vi "Init Nav Panels.vi"(8 "error in (no error)":errorcluster, 11 "App in":refnum<class "App.lvclass">) -> (0 "error out":errorcluster, 3 "App out":refnum<class "App.lvclass">)   [LabVIEW 2020, in "PicoG-App.lvlib" / "App.lvclass"]
uses:
  App.lvclass
  <vilib>/IlluminatedG/IG OOPanel/OOPanel/Manager/Manager.lvclass
  AppListPanel/AppListPanel.lvclass
  DeviceListPanel/DeviceListPanel.lvclass
  PlatformListPanel/PlatformListPanel.lvclass
  C:/Program Files (x86)/National Instruments/LabVIEW 2020/vi.lib/IlluminatedG/IG OOPanel/OOPanel/Panel/Panel.lvclass
  C:/dev/Vireo/PicoG/PicoG-App/AppListPanel/AppListPanel.lvclass
  C:/dev/Vireo/PicoG/PicoG-App/PlatformListPanel/PlatformListPanel.lvclass
  C:/dev/Vireo/PicoG/PicoG-App/DeviceListPanel/DeviceListPanel.lvclass
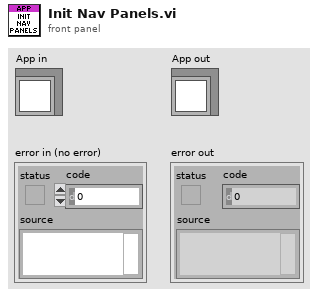
[diagram p1: front panel]
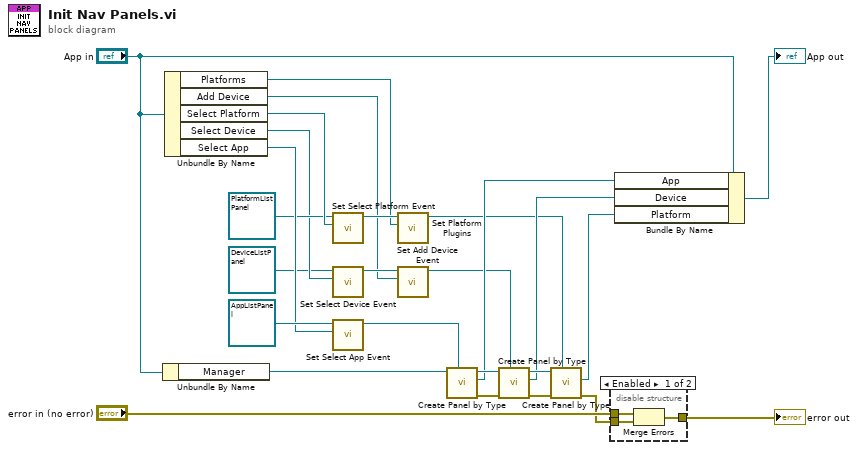
[diagram p0: block diagram]
diagram:
  n1 = Unbundle By Name("App in") -> ("Manager"=w13:refnum<class "Manager.lvclass">)
  n2 = Unbundle By Name("App in") -> ("Platforms"=w1:refnum<class "PlatformPluginManager.lvclass">, "Add Device"=w3:refnum<user-event>, "Select Platform"=w26:refnum<user-event>, "Select Device"=w6:refnum<user-event>, "Select App"=w16:refnum<user-event>)
  n3 = call "Set Select Platform Event.vi"("Select Platform"=w26, "PlatformListPanel in"=refnum<class "PlatformListPanel.lvclass"> refnum ("PicoG-App.lvlib:PlatformListPanel.lvclass")) -> ("PlatformListPanel out"=w8:refnum<class "PlatformListPanel.lvclass">)  [unwired: 8 in, 1 out]
  n4 = call "Set Select Device Event.vi"("Select Device"=w6, "DeviceListPanel in"=refnum<class "DeviceListPanel.lvclass"> refnum ("PicoG-App.lvlib:DeviceListPanel.lvclass")) -> ("DeviceListPanel out"=w4:refnum<class "DeviceListPanel.lvclass">)  [unwired: 8 in, 1 out]
  n5 = call "Set Select App Event.vi"("Select App"=w16, "AppListPanel in"=refnum<class "AppListPanel.lvclass"> refnum ("PicoG-App.lvlib:AppListPanel.lvclass")) -> ("AppListPanel out"=w7:refnum<class "AppListPanel.lvclass">)  [unwired: 8 in, 1 out]
  n6 = call "Set Platform Plugins.vi"("Platform Plugins"=w1, "PlatformListPanel in"=w8) -> ("PlatformListPanel out"=w18:refnum<class "PlatformListPanel.lvclass">)  [unwired: 8 in, 1 out]
  n7 = call "Set Add Device Event.vi"("Add Device"=w3, "DeviceListPanel in"=w4) -> ("DeviceListPanel out"=w2:refnum<class "DeviceListPanel.lvclass">)  [unwired: 8 in, 1 out]
  n8 = call <vilib>:"Create Panel by Type.vi"("Panel Type"=w7, "Manager in"=w13) -> ("error out"=w12:errorcluster, "Panel"=w19:refnum<class "AppListPanel.lvclass">, "Manager out"=w24:refnum<class "Manager.lvclass">)  [unwired: 7 in]
  n9 = call <vilib>:"Create Panel by Type.vi"("Panel Type"=w2, "error in (no error)"=w12, "Manager in"=w24) -> ("error out"=w11:errorcluster, "Panel"=w20:refnum<class "DeviceListPanel.lvclass">, "Manager out"=w23:refnum<class "Manager.lvclass">)  [unwired: 6 in]
  n10 = call <vilib>:"Create Panel by Type.vi"("Panel Type"=w18, "error in (no error)"=w11, "Manager in"=w23) -> ("error out"=w9:errorcluster, "Panel"=w21:refnum<class "PlatformListPanel.lvclass">)  [unwired: 6 in, 1 out]
  n11 = disable-structure shown="Enabled" {
    disable-tunnel: "error in (no error)" -> [w29 w30]
    disable-tunnel: [w28 w30] -> w10
    disable-tunnel: w9 -> [w27 _]
    frame Enabled {
      n12 = Merge Errors(w29, w27) -> (w28:errorcluster)
    }
    frame Disabled {
    }
  }
  "error out" <- w10
  n13 = Bundle By Name(cluster="App in", "App"=w19, "Device"=w20, "Platform"=w21) -> (→"App out":refnum<class "App.lvclass">)
